vi "p1230 write port.vi"(8 "error in (no error)":errorcluster, 10 "data":u32, 11 "board_id":u32) -> (0 "error out":errorcluster, 3 "function return":u32)   [LabVIEW 2014]
doc: "unsigned int __stdcall p1230_write_port(unsigned int board_id, unsigned int data);"
uses:
  PCI1230UTIL.dll
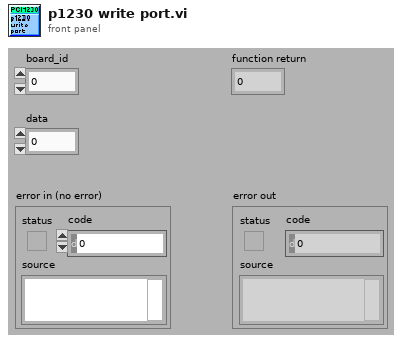
[diagram p1: front panel]
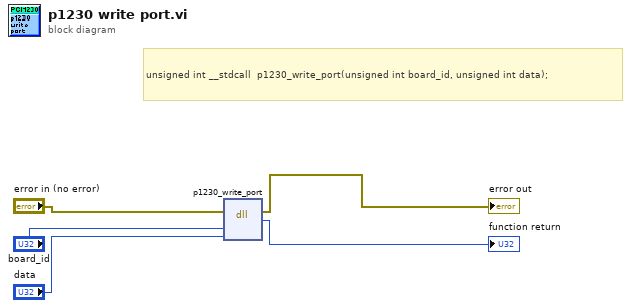
[diagram p0: block diagram]
diagram:
  # "unsigned int __stdcall  p1230_write_port(unsigned int board_id, unsigned int data);"
  n1 = dll-call lib="C:/Users/AICTER/Desktop/PCI-1230/PCI1230_VIs/PCI1230UTIL.*" fn="p1230_write_port"(error in="error in (no error)", "board_id"="board_id", "data"="data") -> (error out=→"error out":errorcluster, "返回类型"=→"function return":u32)  [unwired: 4 in, 1 out]
